vi "Write Icon.vi"(8 "error in (no error)":errorcluster, 9 "Char":T1, 11 "Character LCD in":refnum<class "LEDMatrix.lvclass">) -> (0 "error out":errorcluster, 3 "Character LCD out":refnum<class "LEDMatrix.lvclass">)   [LabVIEW 2020, in "CTI-Peripheral.lvlib" / "LEDMatrix.lvclass"]
uses:
  LEDMatrix.lvclass
  Data Types/ICONS.ctl
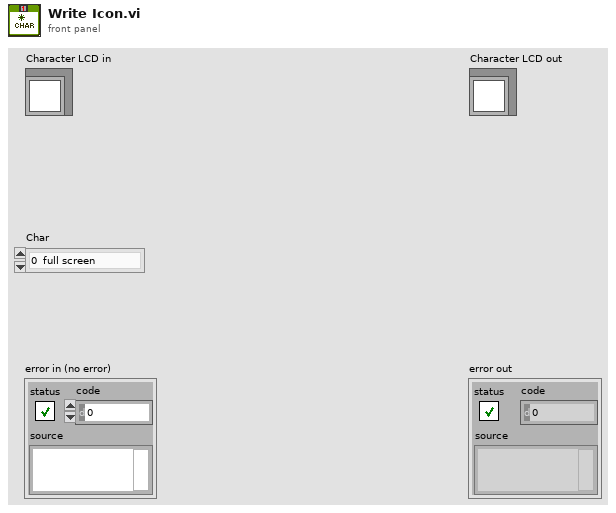
[diagram p1: front panel]
types:
  T1 = typedef "CTI-Peripheral.lvlib/LEDMatrix.lvclass/ICONS.ctl" = enum16{"0  full screen", "1  arrow_up", "2  arrow_down", "3  arrow_right", "4  arrow_left", "5  triangle_up", "6  triangle_down", "7  triangle_right", "8  triangel_left", "9  smile_face_1", "10 smile_face_2", "11 hearts", "12 diamonds", "13 clubs", "14 spades", "15 circle1", "16 circle2", "17 circle3", "18 circle4", "19 man", "20 woman", "21 musical_note_1", "22 musical_note_2", "23 snow", "24 up_down", "25 double_!", "26 left_right", "27 house"}
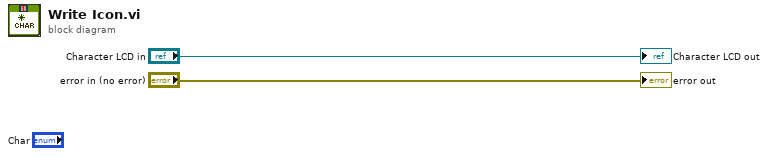
[diagram p0: block diagram]
diagram:
  "error out" <- "error in (no error)"
  "Character LCD out" <- "Character LCD in"
